vi "func_savedata.vi"(8 "append to file? (new file:F)":bool, 9 "1D data":dbl[](array[numeric]), 11 "file path (dialog if empty)":path) -> ()   [LabVIEW 2018]
uses:
  <vilib>/Utility/file.llb/Write Delimited Spreadsheet (DBL).vi
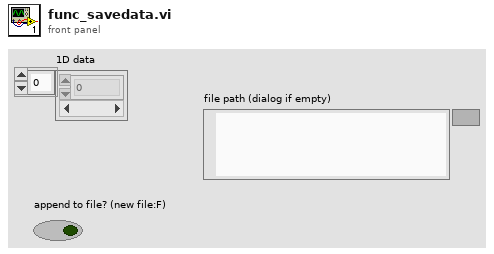
[diagram p1: front panel]
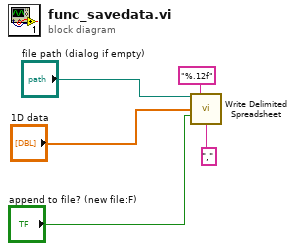
[diagram p0: block diagram]
diagram:
  n1 = call-poly <vilib>:"Write Delimited Spreadsheet.vi"("file path (dialog if empty)"="file path (dialog if empty)", "format (%.3f)"="%.12f", "1D data"="1D data", "append to file? (new file:F)"="append to file? (new file:F)", "delimiter (\\t)"="," ("delimiter (\\t)")) -> ()  [unwired: 9 in, 2 out]
